vi "External Sensor Fudge.vi"(9 "External In":dbl[](array[numeric]), 10 "Commands":dbl[](array[numeric])) -> (2 "External Out":dbl[](array[numeric]))   [LabVIEW 2013]
uses:
  Data Access Objects/Metadata/Persistant DAO Actions.ctl
  Data Access Objects/Application/Number Of LBCBs.ctl
panel:
  in  "Mapping":i32[](array[numeric])=[0, 0, 1, 2, 2, 2, 6, 6, 7, 8, 8, 8]
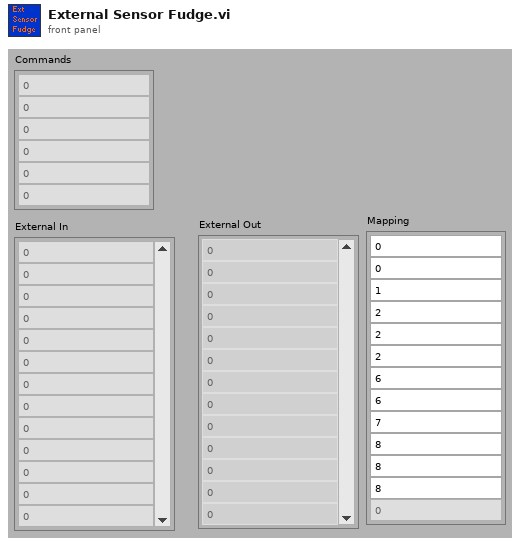
[diagram p1: front panel]
types:
  T1 = typedef "Number Of LBCBs.ctl" = enum16{"1", "2"}
  T2 = typedef "Persistant DAO Actions.ctl" = enum16{"Init", "Get", "Set", "Load", "Save"}
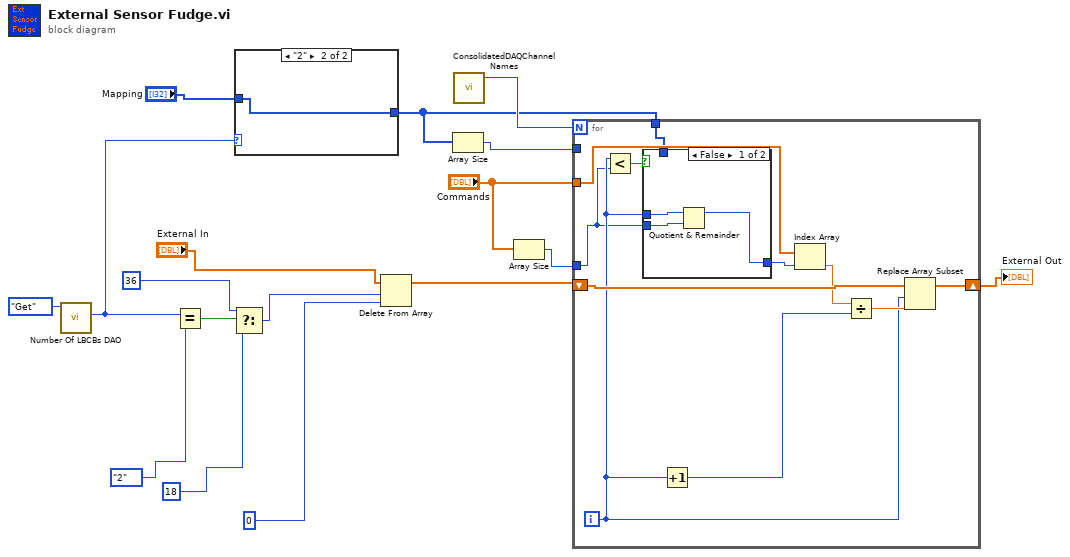
[diagram p0: block diagram]
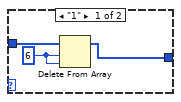
[diagram p2: hidden frame]
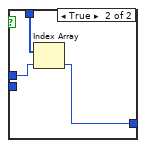
[diagram p3: hidden frame]
diagram:
  n1 = call "Number Of LBCBs DAO.vi"("Actions"=Persistant_DAO_Actions."Get") -> ("Number of\nLBCBs Out"=w4:T1)  [unwired: 4 in, 6 out]
  n2 = Equal?(x=w4, y=Number_Of_LBCBs."2") -> (x = y?=w11:bool)
  n3 = Select(t=36 ("index"), s=w11, f=18) -> (s? t:f=w8:i32)
  n4 = case shown="\"2\"" w4 {
    tunnel: "Mapping" -> [w20 w21]
    tunnel: [w18 w21] -> w2
    frame "1" {
      w19 = 6 ("length")
      n5 = Delete From Array(array=w20, length=w19, index=w19) -> (array with subset deleted=w18:i32[])  [unwired: 1 out]
    }
    frame "2" {
    }
  }
  n6 = Delete From Array(array="External In", length=w8, index=0) -> (array with subset deleted=w14:dbl[])  [unwired: 1 out]
  n7 = Array Size(array=w2) -> (size(s)=w1:i32)
  n8 = call "ConsolidatedDAQChannelNames.vi"() -> ("Number of \nExternal \nChannels 1"=w7:i32)  [unwired: 5 out]
  n9 = Array Size(array="Commands") -> (size(s)=w5:i32)
  n10 = for {
    N: w7 -> [_]
    tunnel: "Commands" -> [w32]
    shift-right: [w30] -> w17
    shift-left: w14 -> [w31]
    tunnel: w5 -> [w22]
    tunnel: w2 -> [w23]
    tunnel: w1 -> [_]
    i -> [w24]
    n11 = Less?(x=w24, y=w22) -> (x < y?=w25:bool)
    n12 = case shown="False" w25 {
      tunnel: [w35 w36] -> w29
      tunnel: w22 -> [w34 _]
      tunnel: w24 -> [w33 w37]
      tunnel: w23 -> [_ w38]
      frame False {
        n13 = Quotient & Remainder(x=w33, y=w34) -> (x-y*floor(x/y)=w35:i32)  [unwired: 1 out]
      }
      frame True {
        n14 = Index Array(array=w38, index=w37) -> (element=w36:i32)
      }
    }
    n15 = Increment(x=w24) -> (x+1=w26:i32)
    n16 = Index Array(array=w32, index=w29) -> (element=w27:dbl)
    n17 = Divide(x=w27, y=w26) -> (x/y=w28:dbl)
    n18 = Replace Array Subset(array=w31, new element=w28, index=w24) -> (w30:dbl[])
  }
  "External Out" <- w17
